vi "Programmatically Manipulate a Tab Control.vi"() -> ()   [LabVIEW 2015]
doc: "Shows how to programmatically manipulate the appearance of a tab control. Specific examples include changing the names of the pages, changing the page enabled state, hiding pages, and coloring individual pages different colors."
panel:
  in  "Hide Page 2?":bool
  in  "Page 2 State":u16(ring) items=["Enabled", "Disabled", "Disabled and Grayed Out"]
  in  "Page 1 State":u16(ring) items=["Enabled", "Disabled", "Disabled and Grayed Out"]
  in  "Page 2 Color":u32(colorbox)=16777215
  in  "Page 1 Color":u32(colorbox)=16750592
  in  "Update Colors":bool
  in  "Update Captions":bool
  in  "Shared Button":bool
  in  "Page 2 Caption":string="Second Page"
  in  "Page 1 Caption":string="First Page"
  in  "Stop":bool
  in  "Tab Control":enum32{"First Page", "Second Page"}(tab)
  in  "Knob":dbl(knob) scale=0.0..10.0
  out "Tank":dbl(slide) scale=0.0..10.0
  out "Waveform Chart":dbl(graph)
  # "Overview: Demonstrates the use of property nodes  to programmatically change the appearance of a Tab Control.\nInstructions:\n1. Run the VI.\n2. Click Update Captions to update the caption text on each tab.\n3. Click Update Colors to change the colors of each tab.\n4. Change the Page 1 State and Page 2 State values to enable and disable pages.\n5. Click the Hide Page 2? button to hide and show the second page.\n6. Click Stop to stop the VI."
  # "To see the right-click menu for the tab control, you must click on its border."
  # "Note: The Shared Button is visible on all pages of the tab control. This is because it was dropped on the panel and moved over the tab control, as opposed to being dropped within the tab control itself. The shadow under the control disappears when the VI runs."
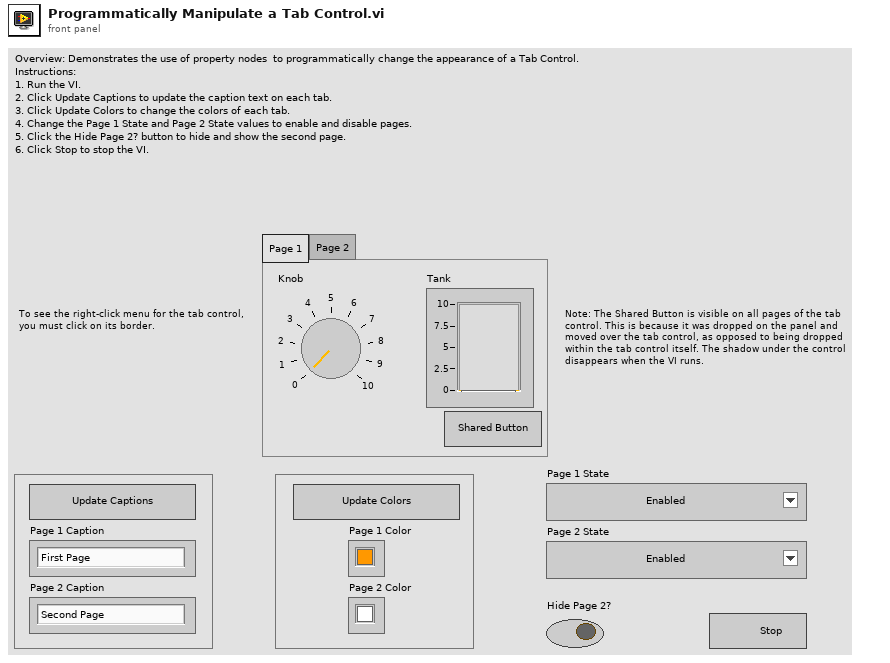
[diagram p1: front panel]
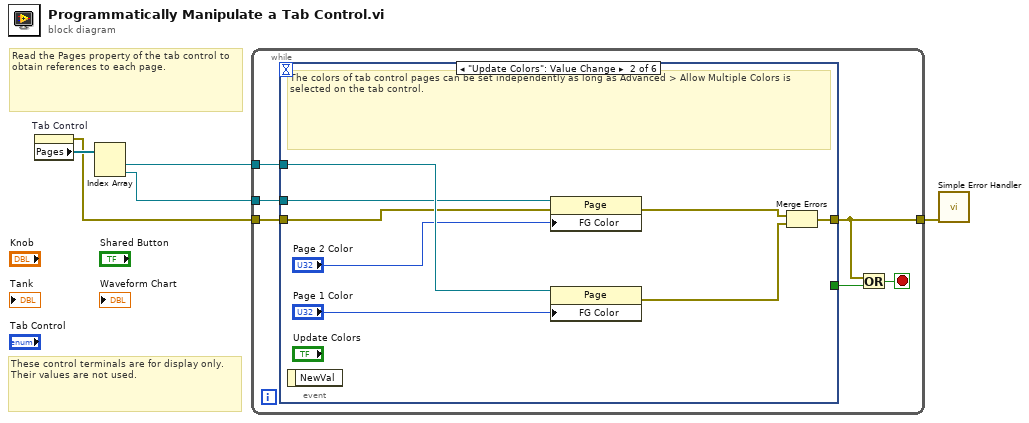
[diagram p0: block diagram]
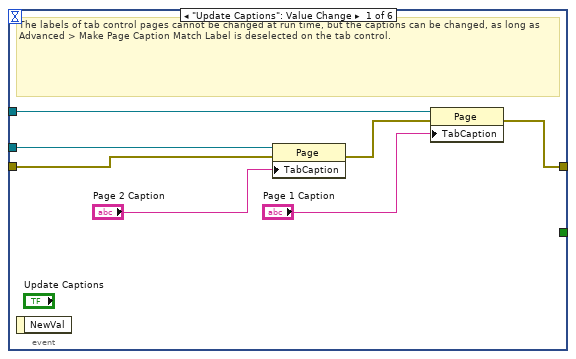
[diagram p2: hidden frame]
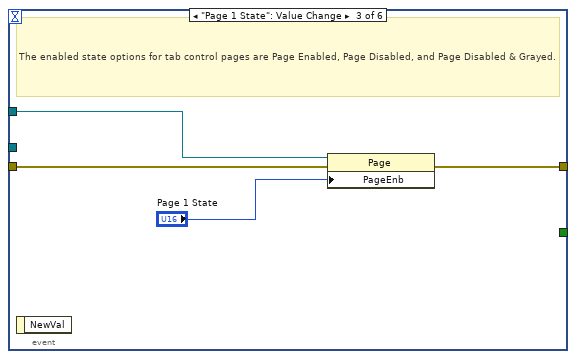
[diagram p3: hidden frame]
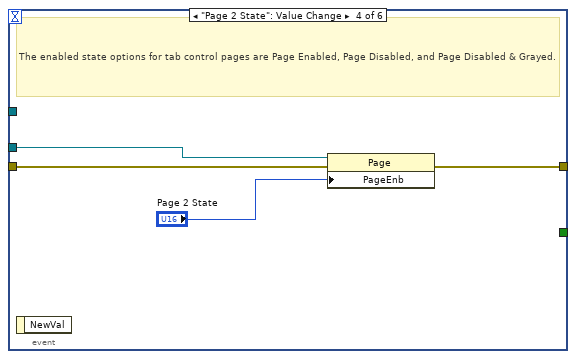
[diagram p4: hidden frame]
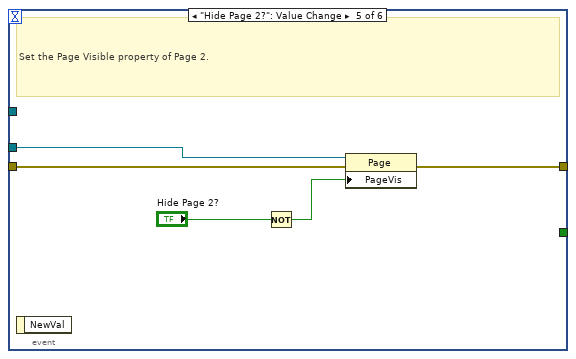
[diagram p5: hidden frame]
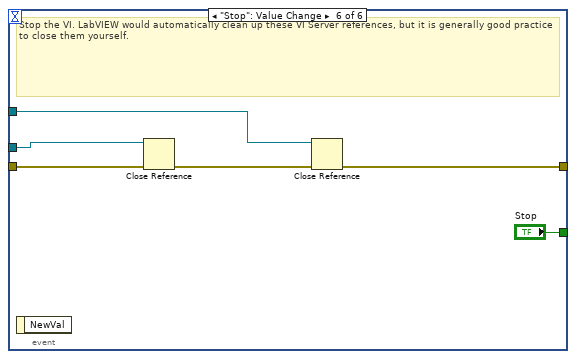
[diagram p6: hidden frame]
diagram:
  # "These control terminals are for display only. Their values are not used."
  # "Read the Pages property of the tab control to obtain references to each page."
  n1 = property on="Tab Control" class="TabCtl (strict)"() -> (error out=w2:errorcluster, "Pages"=w5:refnum<vi>[])  [unwired: 2 in, 1 out]
  n2 = Index Array(array=w5) -> (element #1=w4:refnum<vi>, element #2=w3:refnum<vi>)  [unwired: 2 in]
  n3 = while {
    tunnel: w4 -> [w10]
    tunnel: w3 -> [w9]
    tunnel: w2 -> [w8]
    tunnel: [w6] -> w1
    stop <- w7 stop-if-true
    n4 = event shown="[1] \"Update Colors\": Value Change" {
      selector: _ -> [_ _ _ _ _ _]
      dyn-events: _ -> [_ _ _ _ _ _]
      timeout: _ -> [_ _ _ _ _ _]
      tunnel: [_ _ _ _ _ "Stop"] -> w11
      tunnel: w10 -> [w18 w26 w27 _ _ w40]
      tunnel: w9 -> [w17 w25 _ w34 w39 w41]
      tunnel: w8 -> [w16 w24 w30 w33 w38 w44]
      tunnel: [w14 w19 w29 w32 w37 w42] -> w6
      event "Update Captions": Value Change {
        # "The labels of tab control pages cannot be changed at run time, but the captions can be changed, as long as Advanced > Make Page Caption Match Label is deselected on the tab control."
        n5 = event-data() -> ()  [unwired: 1 in, 1 out]
        n6 = property class="Page"(reference=w17, error in=w16, "TabCaption"="Page 2 Caption") -> (error out=w15:errorcluster)  [unwired: 1 out]
        n7 = property class="Page"(reference=w18, error in=w15, "TabCaption"="Page 1 Caption") -> (error out=w14:errorcluster)  [unwired: 1 out]
      }
      event "Update Colors": Value Change {
        # "The colors of tab control pages can be set independently as long as Advanced > Allow Multiple Colors is selected on the tab control."
        n8 = event-data() -> ()  [unwired: 1 in, 1 out]
        n9 = property class="Page"(reference=w25, error in=w24, "FG Color"="Page 2 Color") -> (error out=w21:errorcluster)  [unwired: 1 out]
        n10 = property class="Page"(reference=w26, "FG Color"="Page 1 Color") -> (error out=w20:errorcluster)  [unwired: 1 in, 1 out]
        n11 = Merge Errors(w21, w20) -> (w19:errorcluster)
      }
      event "Page 1 State": Value Change {
        # "The enabled state options for tab control pages are Page Enabled, Page Disabled, and Page Disabled & Grayed."
        n12 = event-data() -> ()  [unwired: 1 in, 1 out]
        n13 = property class="Page"(reference=w27, error in=w30, "PageEnb"="Page 1 State") -> (error out=w29:errorcluster)  [unwired: 1 out]
      }
      event "Page 2 State": Value Change {
        # "The enabled state options for tab control pages are Page Enabled, Page Disabled, and Page Disabled & Grayed."
        n14 = event-data() -> ()  [unwired: 1 in, 1 out]
        n15 = property class="Page"(reference=w34, error in=w33, "PageEnb"="Page 2 State") -> (error out=w32:errorcluster)  [unwired: 1 out]
      }
      event "Hide Page 2?": Value Change {
        # "Set the Page Visible property of Page 2."
        n16 = event-data() -> ()  [unwired: 1 in, 1 out]
        n17 = Not(x="Hide Page 2?") -> (.not. x?=w35:bool)
        n18 = property class="Page"(reference=w39, error in=w38, "PageVis"=w35) -> (error out=w37:errorcluster)  [unwired: 1 out]
      }
      event "Stop": Value Change {
        # "Stop the VI. LabVIEW would automatically clean up these VI Server references, but it is generally good practice to close them yourself."
        n19 = event-data() -> ()  [unwired: 1 in, 1 out]
        n20 = Close Reference(reference=w41, error in (no error)=w44) -> (error out=w43:errorcluster)
        n21 = Close Reference(reference=w40, error in (no error)=w43) -> (error out=w42:errorcluster)
      }
    }
    n22 = Or(x=w6, y=w11) -> (x .or. y?=w7:bool)
  }
  n23 = call <vilib>:"Simple Error Handler.vi"("error in (no error)"=w1) -> ()  [unwired: 4 in, 5 out]
